vi "checkFinishKickPenaltyAllyPlay.vi"(8 "error in (no error)":errorcluster, 10 "Game":refnum<class "Game.lvclass">, 11 "KickPenaltyAllyPlay in":refnum<class "KickPenaltyAllyPlay.lvclass">) -> (0 "error out":errorcluster, 2 "Boolean":bool, 3 "KickPenaltyAllyPlay out":refnum<class "KickPenaltyAllyPlay.lvclass">)   [LabVIEW 2023, in "KickPenaltyAllyPlay.lvclass"]
uses:
  KickPenaltyAllyPlay.lvclass
  Game_class/Game.lvclass
  Referee_class/command_interpreted.ctl
  Game_class/Game.lvclass/Game.ctl
  Referee_class/Referee.lvclass/Referee.ctl
  Events_class/Events.lvclass/Events.ctl
  Game_class/Read Referee.vi
  Game_class/Read EventsRef.vi
  Events_class/Read ball_out.vi
  Events_class/Read touch.vi
  Events_class/Read ball_out_of_vision.vi
  Events_class/Read id_touch.vi
  Referee_class/Read command_interpreted.vi
  Referee_class/Referee.lvclass
  Events_class/Events.lvclass
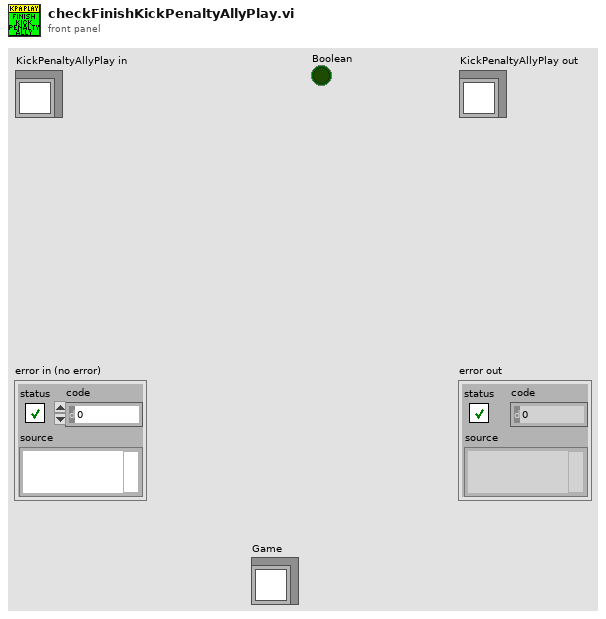
[diagram p1: front panel]
types:
  T1 = typedef "command_interpreted.ctl" = enum16{"Goal Ally", "Goal Enemy", "Ball Placement Enemy", "Ball Placement Ally", "Normal Half Time", "Extra Time  Break", "Extra Half Time", "None", "Post Game", "PKA Normal Start", "Prepare Kickoff Ally", "PKE Normal Start", "Prepare Kickoff Enemy", "Force Start", "Halt", "Timeout", "Prepare Penalty Ally", "Prepare Penalty Enemy", "PPA NormalStart", "PPE Normal Start", "Indirect Free Ally", "Direct Free Enemy", "Direct Free Ally", "Indirect Free Enemy", "Stop"}
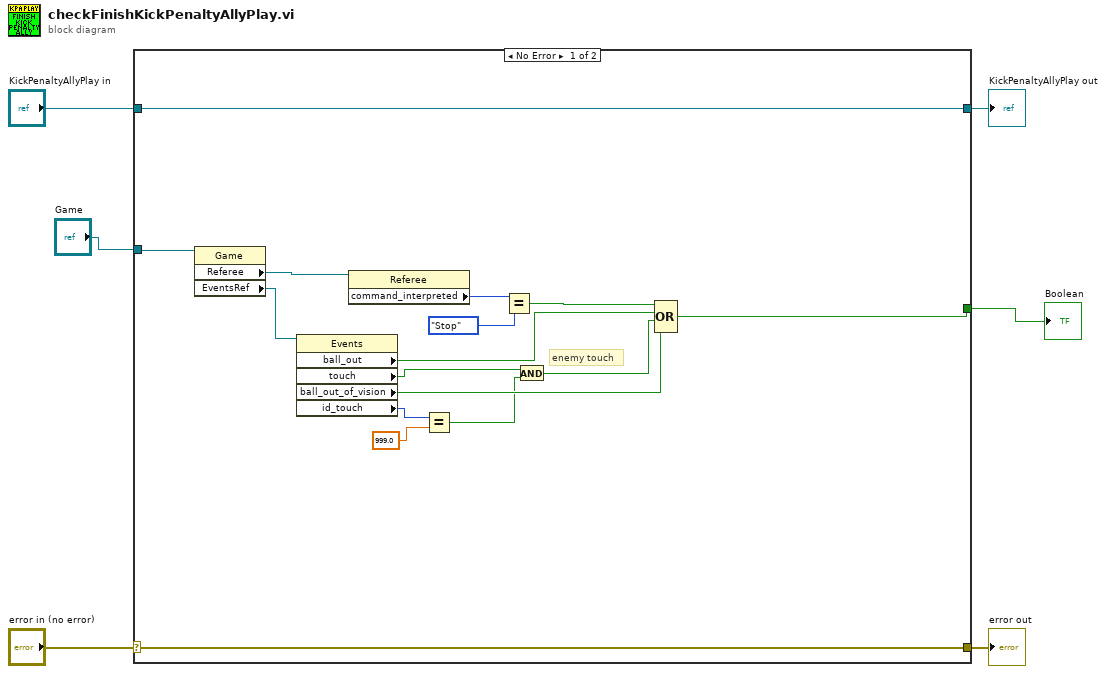
[diagram p0: block diagram]
diagram:
  n1 = case shown="No Error" "error in (no error)" {
    selector: "error in (no error)" -> [w21 w24]
    tunnel: [w21 w24] -> w5
    tunnel: [w22 w23] -> w3
    tunnel: "KickPenaltyAllyPlay in" -> [w22 w23]
    tunnel: "Game" -> [w18 _]
    tunnel: [w15 _] -> w1
    frame No Error {
      # "enemy touch"
      n2 = property class="Game"(reference=w18) -> ("Referee"=w20:refnum<class "Referee.lvclass">, "EventsRef"=w17:refnum<class "Events.lvclass">)  [unwired: 1 in, 2 out]
      n3 = property class="Events"(reference=w17) -> ("ball_out"=w16:bool, "touch"=w12:bool, "ball_out_of_vision"=w14:bool, "id_touch"=w11:i32)  [unwired: 1 in, 2 out]
      n4 = property class="Referee"(reference=w20) -> ("command_interpreted"=w19:T1)  [unwired: 1 in, 2 out]
      n5 = Equal?(x=w11, y=999.0) -> (x = y?=w9:bool)
      n6 = Equal?(x=w19, y=command_interpreted."Stop") -> (x = y?=w7:bool)
      n7 = And(x=w12, y=w9) -> (x .and. y?=w13:bool)
      n8 = Compound Arithmetic op=OR(w7, w16, w13, w14) -> (w15:bool)
    }
    frame Error {
    }
  }
  "error out" <- w5
  "KickPenaltyAllyPlay out" <- w3
  "Boolean" <- w1
